vi "质控单元MB_api.vi"(6 "Slave ID":u8=1, 7 "STEP":enum16{"open", "read", "write", "close"}(ring)=enum."read", 8 "Error in":errorcluster caption="Error in (no error)", 9 "values":u16[](array[numeric]), 10 "quantity":u16, 11 "starting address":u16 format="%04xH") -> (0 "error out":errorcluster, 1 "MB session out":refnum<class "MB_Master.lvclass">, 2 "MB_TCP session":refnum<class "MB_Master_TCP.lvclass">, 3 "Registers":u16[](array[numeric]))   [LabVIEW 2016, in "质控单元.lvlib"]
uses:
  <vilib>/Plasmionique/MB Master/MB_Master/MB_Master.lvclass
  <vilib>/Plasmionique/MB Master/MB_Master_TCP/MB_Master_TCP.lvclass
  D:/Program Files (x86)/National Instruments/LabVIEW 2016/vi.lib/Plasmionique/MB Master/MB_Master/MB_Master.lvclass
  <vilib>/Plasmionique/MB Master/MB_Master_Serial/MB_Master_Serial.lvclass
  <vilib>/Plasmionique/MB Master/MB Master.lvlib
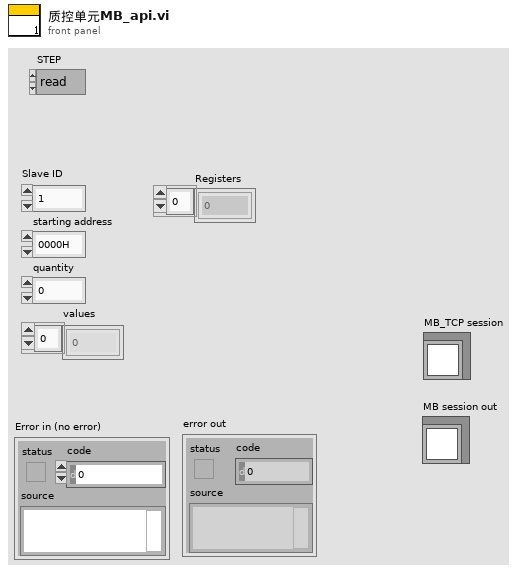
[diagram p1: front panel]
types:
  T1 = cluster{"baud rate (bps)":u32, "stop bits":u16, "parity":u16, "flow control":u16, "timeout":u32, "retries":i32}
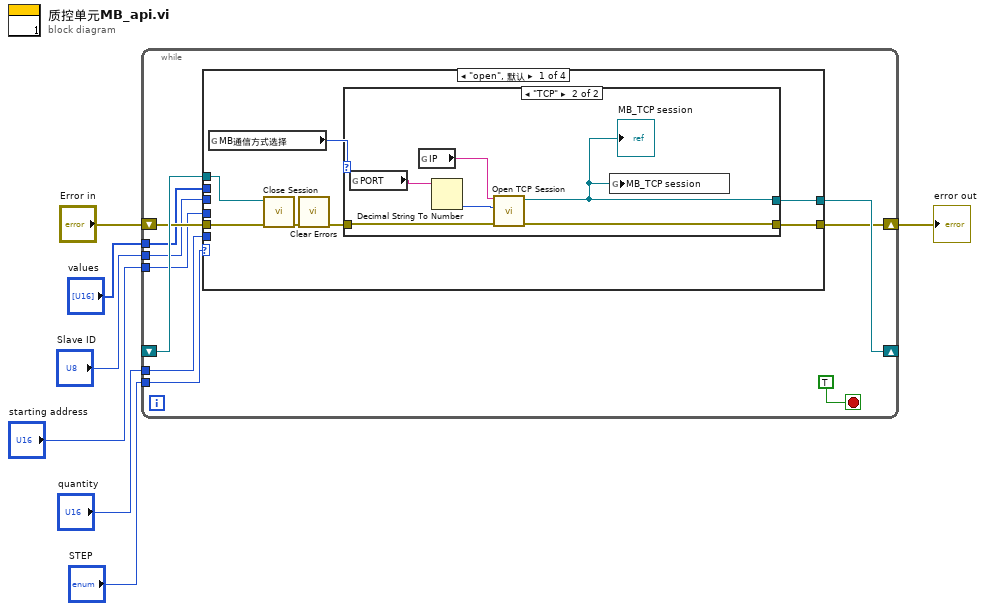
[diagram p0: block diagram]
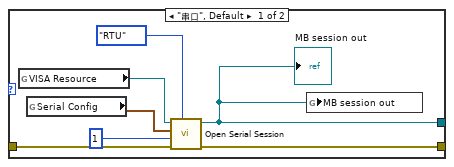
[diagram p2: hidden frame]
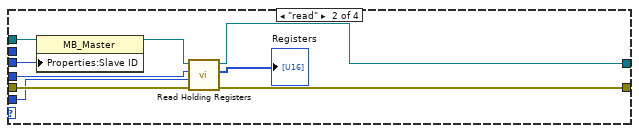
[diagram p3: hidden frame]
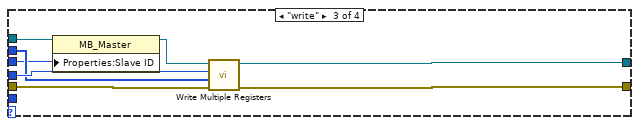
[diagram p4: hidden frame]
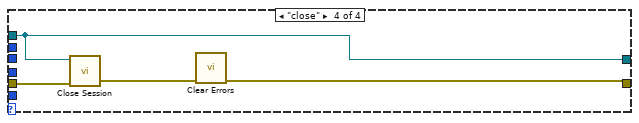
[diagram p5: hidden frame]
diagram:
  n1 = while {
    shift-right: [w11] -> _
    shift-left: _ -> [w17]
    shift-right: [w10] -> w6
    shift-left: "Error in" -> [w16]
    tunnel: "Slave ID" -> [w15]
    tunnel: "starting address" -> [w14]
    tunnel: "quantity" -> [w13]
    tunnel: "STEP" -> [w12]
    tunnel: "values" -> [w9]
    stop <- TRUE stop-if-true
    n2 = case shown="\"open\", 默认" w12 {
      tunnel: w17 -> [w22 w39 w49 w57]
      tunnel: w16 -> [w21 w46 w54 w58]
      tunnel: [w23 w45 w52 w57] -> w11
      tunnel: [w24 w44 w53 w55] -> w10
      tunnel: w15 -> [_ w42 w48 _]
      tunnel: w14 -> [_ w41 w51 _]
      tunnel: w13 -> [_ w40 _ _]
      tunnel: w9 -> [_ _ w50 _]
      frame "open", Default {
        n3 = global read "断电保存全局.vi" "MB通信方式选择"() -> (w18:enum16{"串口", "TCP"})
        n4 = call-dynamic "Close Session.vi"("error in (no error)"=w21, "MB session in"=w22) -> ("error out"=w20:errorcluster)  [unwired: 9 in]
        n5 = call <vilib>:"Clear Errors.vi"("error in (no error)"=w20) -> ("error out"=w19:errorcluster)  [unwired: 5 in, 1 out]
        n6 = case shown="\"TCP\"" w18 {
          tunnel: [w30 w34] -> w24
          tunnel: [w26 w32] -> w23
          tunnel: w19 -> [w27 w33]
          frame "串口", Default {
            n7 = global read "断电保存全局.vi" "VISA Resource"() -> (w29:refnum<visa-resource-name>)
            n8 = global read "断电保存全局.vi" "Serial Config"() -> (w28:T1)
            n9 = call <vilib>:"Open Serial Session.vi"("Mode (RTU)"=enum16{"RTU", "ASCII"}."RTU", "Error in"=w27, "Slave ID"=u8 1, "Serial Config"=w28, "VISA Resource"=w29) -> ("Error out"=w30:errorcluster, "MB_Serial session"=w26:refnum<class "MB_Master_Serial.lvclass">)  [unwired: 5 in]
            "MB session out" <- w26
            n10 = global write "断电保存全局.vi" "MB session out"(w26) -> ()
          }
          frame "TCP" {
            n11 = global read "断电保存全局.vi" "PORT"() -> (w36:string)
            n12 = global read "断电保存全局.vi" "IP"() -> (w35:string)
            n13 = Decimal String To Number(string=w36) -> (number=w37:i32)  [unwired: 2 in, 1 out]
            n14 = call <vilib>:"Open TCP Session.vi"("error in (no error)"=w33, "Port (502)"=w37, "IP Address"=w35) -> ("error out"=w34:errorcluster, "MB_TCP session"=w32:refnum<class "MB_Master_TCP.lvclass">)  [unwired: 7 in]
            "MB_TCP session" <- w32
            n15 = global write "断电保存全局.vi" "MB_TCP session"(w32) -> ()
          }
        }
      }
      frame "read" {
        n16 = property class="MB_Master"(reference=w39, "Properties:Slave ID"=w42) -> (reference out=w38:refnum<class "MB_Master.lvclass">)  [unwired: 1 in, 1 out]
        n17 = call <vilib>:"Read Holding Registers.vi"("error in (no error)"=w46, "quantity"=w40, "starting address"=w41, "MB session in"=w38) -> ("error out"=w44:errorcluster, "Registers"=→"Registers":u16[], "MB session out"=w45:refnum<class "MB_Master.lvclass">)  [unwired: 5 in]
      }
      frame "write" {
        n18 = property class="MB_Master"(reference=w49, "Properties:Slave ID"=w48) -> (reference out=w47:refnum<class "MB_Master.lvclass">)  [unwired: 1 in, 1 out]
        n19 = call <vilib>:"Write Multiple Registers.vi"("error in (no error)"=w54, "values"=w50, "starting address"=w51, "MB session in"=w47) -> ("error out"=w53:errorcluster, "MB session out"=w52:refnum<class "MB_Master.lvclass">)  [unwired: 6 in]
      }
      frame "close" {
        n20 = call-dynamic "Close Session.vi"("error in (no error)"=w58, "MB session in"=w57) -> ("error out"=w56:errorcluster)  [unwired: 9 in]
        n21 = call <vilib>:"Clear Errors.vi"("error in (no error)"=w56) -> ("error out"=w55:errorcluster)  [unwired: 5 in, 1 out]
      }
    }
  }
  "error out" <- w6
